vi "Robot Main.vi"() -> ()   [LabVIEW 2023]
doc: "This VI implements the framework and scheduler for your robotics program. It should not be necessary to modify the framework. You are expected to add your code to the VIs called from Robot Main - the ones located in the Team Code folder within the project."
uses:
  <vilib>/Rock Robotics/WPI/Camera/WPI_CameraImageSize.ctl
  RoboRIO Utilities/Global_STOP.vi
  Robot Global Data.vi
panel:
  in  "Image Size":T1=enum."320x240"
  in  "Enable Vision":bool
  in  "Finish":bool
  # "DRIVER"
  # "COPILOT"
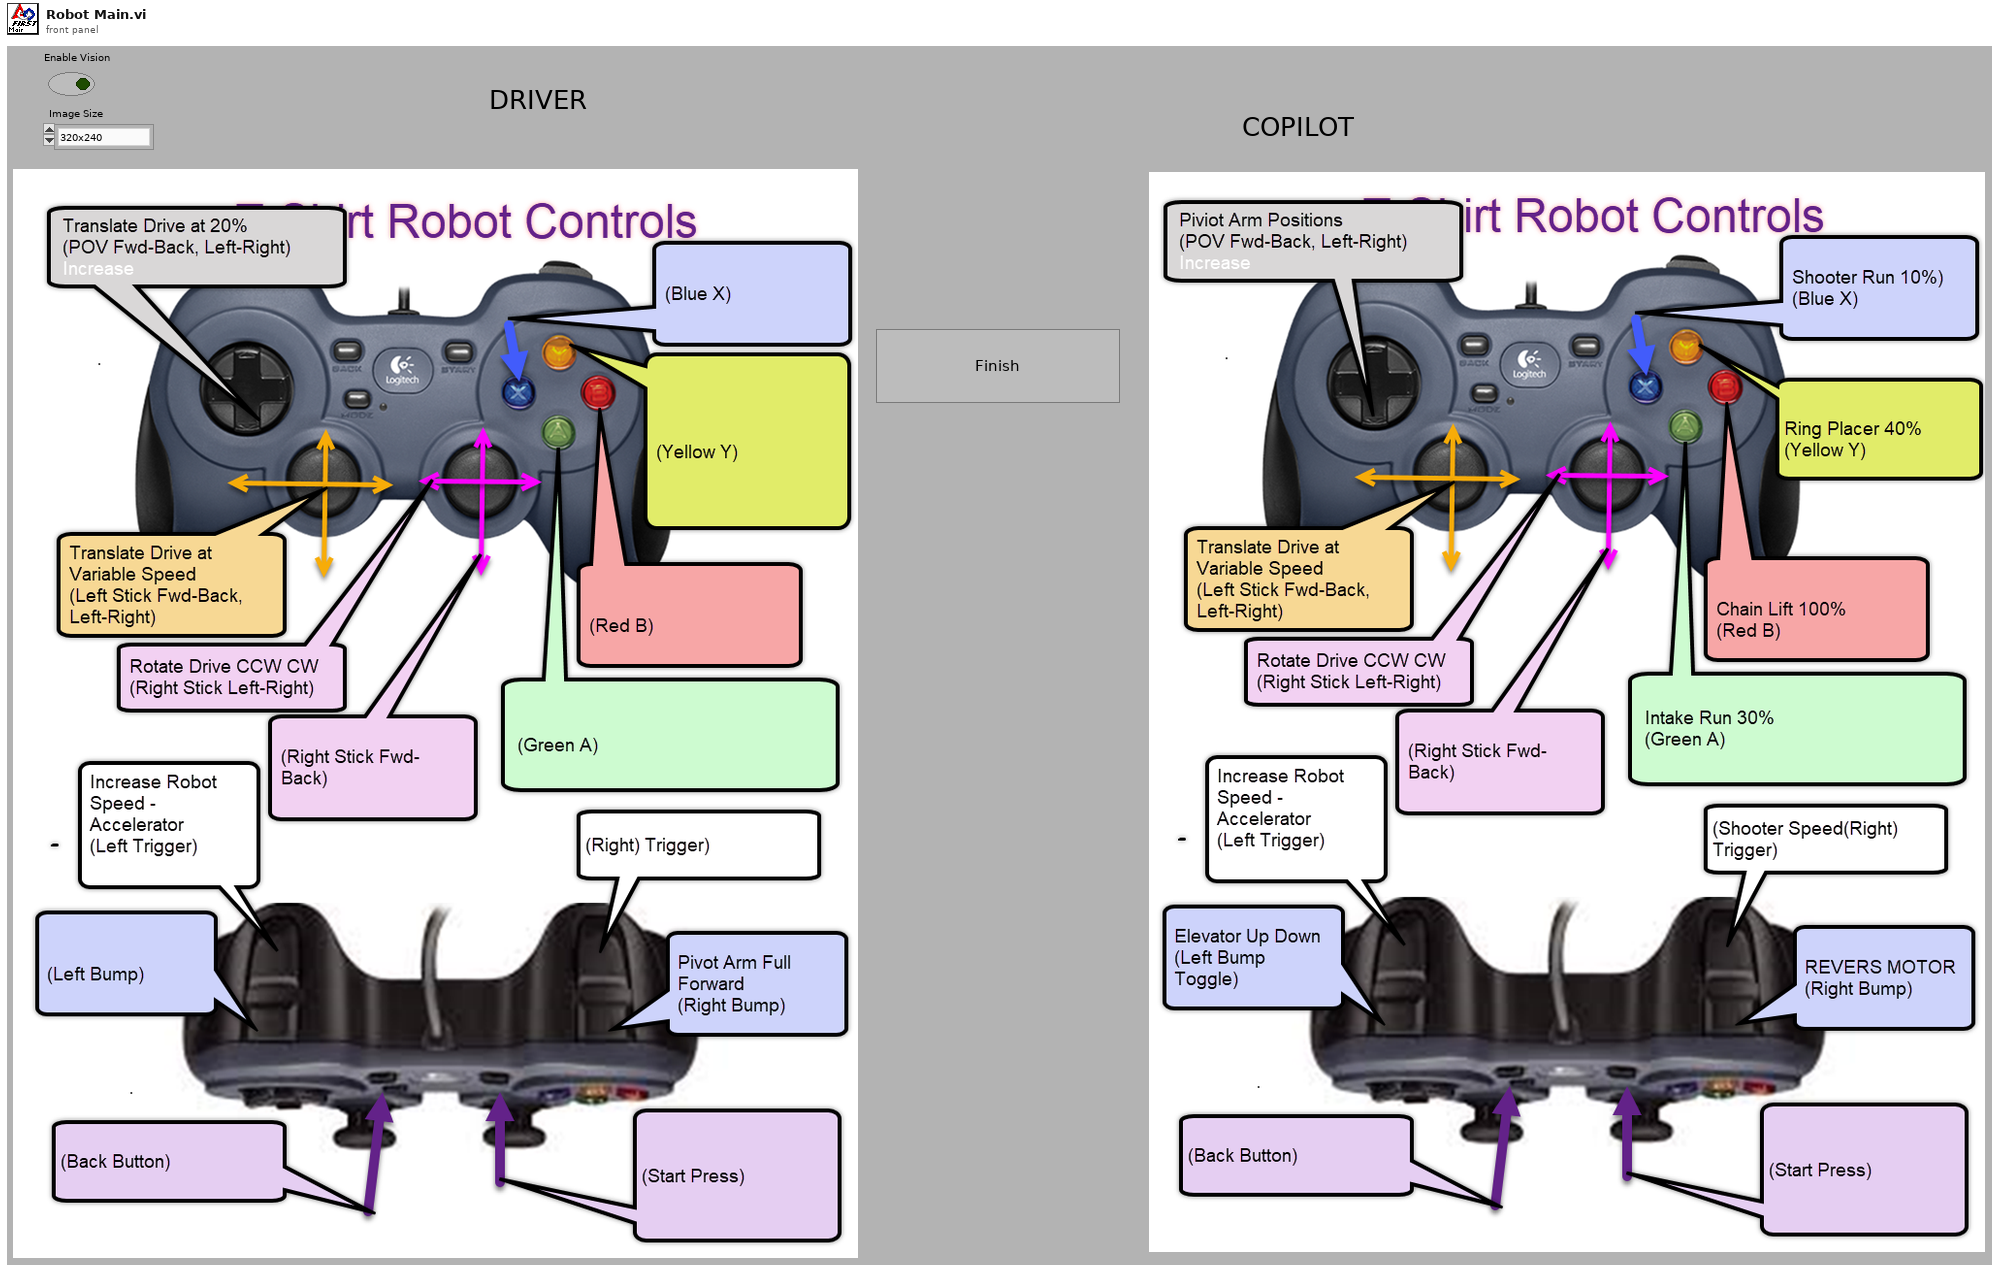
[diagram p1: front panel]
types:
  T1 = typedef "WPI_CameraImageSize.ctl" = enum16{"640x480", "320x240", "160x120", "Custom"}
  T2 = typedef "WPI_DriverStationMatch Info.ctl" = cluster{"Autonomous Elapsed Seconds":dbl, "TeleOp Elapsed Seconds":dbl, "Disabled Elapsed Seconds":dbl, "Visited Autonomous":bool, "Visited TeleOp":bool, "Visited Disabled":bool, "Autonomous Settings":cluster{"Autonomous Style":enum16{"Iterative", "Independent"}, "VI Refnum":refnum<vi>}}
  T3 = typedef "WPI_DriverStationDerivedRobotMode.ctl" = enum16{"Init", "Execute", "Stop"}
  T4 = typedef "WPI_DriverStationRobotMode2.ctl" = enum16{"Autonomous Disabled", "Autonomous Enabled", "Teleop Disabled", "Teleop Enabled", "Disconnected", "Finish", "Test Disabled", "Test Enabled", "Emergency Stopped"}
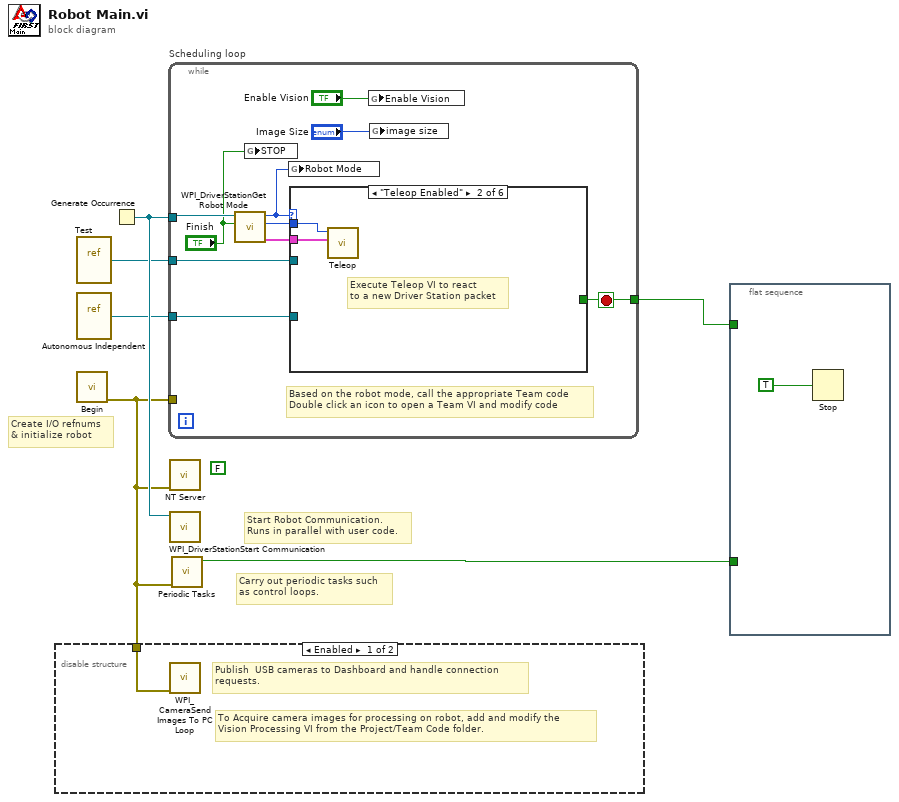
[diagram p0: block diagram]
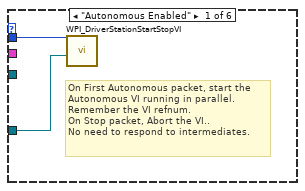
[diagram p3: hidden frame]
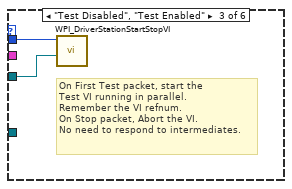
[diagram p4: hidden frame]
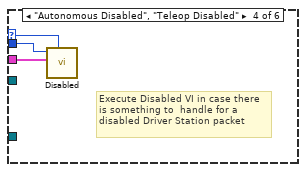
[diagram p5: hidden frame]
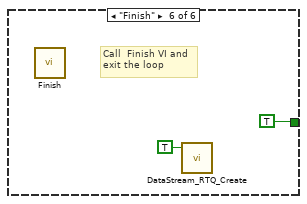
[diagram p7: hidden frame]
diagram:
  (unwired) FALSE
  # "Carry out periodic tasks such\nas control loops."
  # "Create I/O refnums\n& initialize robot"
  # "Start Robot Communication.\nRuns in parallel with user code."
  n1 = vi-ref "Test.vi"() -> (w4:refnum<vi>)
  n2 = vi-ref "Autonomous Independent.vi"() -> (w5:refnum<vi>)
  n3 = call "Begin.vi"() -> ("error out"=w3:errorcluster)  [unwired: 2 in, 9 out]
  n4 = disable-structure shown="Enabled" {
    disable-tunnel: w3 -> [w7 _]
    frame Enabled {
      # "Publish  USB cameras to Dashboard and handle connection\nrequests."
      # "To Acquire camera images for processing on robot, add and modify the\nVision Processing VI from the Project/Team Code folder."
      n5 = call <vilib>:"WPI_CameraSend Images To PC Loop.vi"("error in (no error)"=w7) -> ()  [unwired: 11 in]
    }
    frame Disabled {
    }
  }
  n6 = Generate Occurrence() -> (w6:refnum<k4>)
  n7 = while "Scheduling loop" {
    tunnel: w6 -> [w16]
    tunnel: w3 -> [_]
    tunnel: w5 -> [w13]
    tunnel: w4 -> [w11]
    tunnel: [w8] -> w2
    stop <- w8 stop-if-true
    # "Based on the robot mode, call the appropriate Team code\nDouble click an icon to open a Team VI and modify code"
    n8 = call <vilib>:"WPI_DriverStationGet Robot Mode.vi"("Finish"="Finish", "DS Occurrence"=w16) -> ("Match Info out"=w15:T2, "Call Context"=w17:T3, "Robot Mode"=w10:T4)  [unwired: 7 out]
    n9 = global write "Global_STOP.vi" "STOP"("Finish") -> ()
    n10 = global write "Robot Global Data.vi" "Robot Mode"(w10) -> ()
    n11 = case shown="\"Teleop Enabled\"" w10 {
      selector: w10 -> [_ _ _ w24 _ _]
      tunnel: w17 -> [w19 w21 w23 w26 _ _]
      tunnel: w15 -> [_ w20 _ w25 _ _]
      tunnel: [_ _ _ _ _ TRUE] -> w8
      tunnel: w13 -> [w18 _ _ _ _ _]
      tunnel: w11 -> [_ _ w22 _ _ _]
      frame "Autonomous Enabled" {
        # "On First Autonomous packet, start the\nAutonomous VI running in parallel.\nRemember the VI refnum.\nOn Stop packet, Abort the VI..\nNo need to respond to intermediates."
        n12 = call <vilib>:"WPI_DriverStationStartStopVI.vi"("VI in"=w18, "Call Context"=w19) -> ()  [unwired: 10 in]
      }
      frame "Teleop Enabled" {
        # "Execute Teleop VI to react\nto a new Driver Station packet"
        n13 = call "Teleop.vi"("Match Info"=w20, "Call Context"=w21) -> ()  [unwired: 1 in, 9 out]
      }
      frame "Test Disabled", "Test Enabled" {
        # "On First Test packet, start the\nTest VI running in parallel.\nRemember the VI refnum.\nOn Stop packet, Abort the VI.\nNo need to respond to intermediates."
        n14 = call <vilib>:"WPI_DriverStationStartStopVI.vi"("VI in"=w22, "Call Context"=w23) -> ()  [unwired: 10 in]
      }
      frame "Autonomous Disabled", "Teleop Disabled" {
        # "Execute Disabled VI in case there\nis something to  handle for a\ndisabled Driver Station packet"
        n15 = call "Disabled.vi"("Robot Mode"=w24, "Match Info"=w25, "Call Context"=w26) -> ()  [unwired: 1 in, 8 out]
      }
      frame "Disconnected", Default {
        # "Driver Station packet didn't arrive.\nPossibly useful for diagnostics"
      }
      frame "Finish" {
        # "Call  Finish VI and\nexit the loop"
        n16 = call "Finish.vi"() -> ()  [unwired: 1 in, 7 out]
        n17 = call "DataStream_RTQ_Create.vi"("Close Queue"=TRUE) -> ()  [unwired: 10 in, 1 out]
      }
    }
    n18 = global write "Robot Global Data.vi" "Enable Vision"("Enable Vision") -> ()
    n19 = global write "Robot Global Data.vi" "image size"("Image Size") -> ()
  }
  n20 = call <vilib>:"NT Server.vi"("error in (no error)"=w3) -> ()  [unwired: 10 in, 1 out]
  n21 = call <vilib>:"WPI_DriverStationStart Communication.vi"("occurrence"=w6) -> ()  [unwired: 2 in, 9 out]
  n22 = call "Periodic Tasks.vi"("error in"=w3) -> ("Boolean"=w1:bool)  [unwired: 1 in, 9 out]
  n23 = flat-sequence {
    tunnel: w2 -> [_]
    tunnel: w1 -> [_]
    frame #0 {
      n24 = Stop(stop? (T)=TRUE ("Quit")) -> ()
    }
  }
